vi "DIMPowerSupply.UpdateVoltage.vi"(0 "i ref in":refnum<vi>, 1 "badValue":bool, 2 "moduleValue":dbl format="%.2f", 3 "ms timeout (10000)":i32=10000, 5 "error in (no error)":errorcluster, 6 "voltageQuality":i32) -> (14 "i ref out":refnum<vi>, 17 "timed out":bool, 19 "error out":errorcluster)   [LabVIEW 2014, in "DIMPowerSupply.lvlib"]
doc: "Takes the inpute (raw) voltage and calcutes the real actual voltage [V] delivered by the power supply.\n\nThe value of the actual voltage is written to the attribute data and published via DIM.\n\nThe bad-status bit is also determined and updated."
uses:
  DIMPowerSupply.lvlib
  CSlibraries/UtilityLib/UtilityLib.valueStatus.ctl
  CS_Core/CSApplicationBaseClasses/PSChannelBase/PSChannelBase.statusType.ctl
  CS_Core/CSApplicationBaseClasses/PSChannelBase/PSChannelBase.directionType.ctl
  CS_Core/CSApplicationBaseClasses/PSChannelBase/PSChannelBase.serviceType.ctl
  CS_Core/CSApplicationBaseClasses/PSChannelBase/PSChannelBase.lvlib
  CSlibraries/UtilityLib/UtilityLib.lvlib
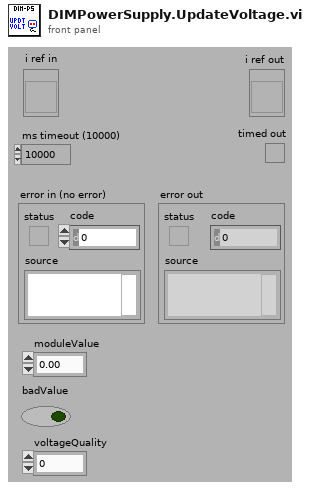
[diagram p1: front panel]
types:
  T1 = typedef "PSChannelBase.lvlib/PSChannelBase.serviceType.ctl" = enum16{"onOff", "voltage", "current", "tripCurrent", "rampUpSpeed", "rampDownSpeed", "status"}
  T2 = typedef "UtilityLib.lvlib/UtilityLib.valueStatus.ctl" = enum16{"no info available", "stand by/off", "on", "warning", "alarm/malfunction", "not implemented", "user action required", "important information", "system default", "control default", "indicator default", "button default"}
  T3 = typedef "PSChannelBase.lvlib/PSChannelBase.directionType.ctl" = enum16{"unknown", "update actual value", "update nominal value", "update both"}
  T4 = typedef "PSChannelBase.lvlib/PSChannelBase.statusType.ctl" = i32
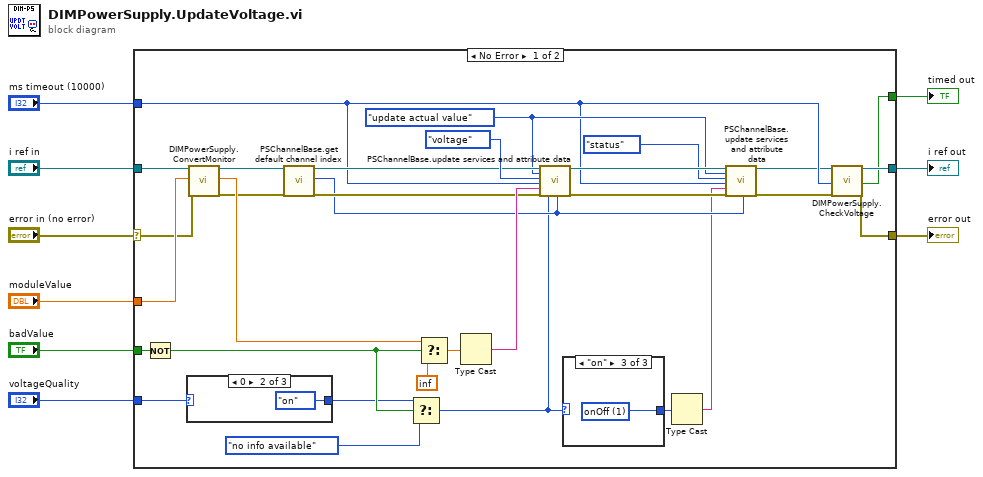
[diagram p0: block diagram]
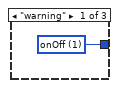
[diagram p2: hidden frame]
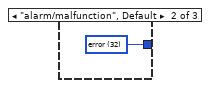
[diagram p3: hidden frame]
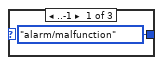
[diagram p4: hidden frame]
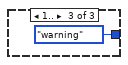
[diagram p5: hidden frame]
diagram:
  n1 = case shown="No Error" "error in (no error)" {
    selector: "error in (no error)" -> [w38 w47]
    tunnel: "i ref in" -> [w40 w48]
    tunnel: "moduleValue" -> [w39 _]
    tunnel: "ms timeout (10000)" -> [w18 _]
    tunnel: [w37 w48] -> w6
    tunnel: [w36 w47] -> w5
    tunnel: [w10 _] -> w4
    tunnel: "badValue" -> [w35 _]
    tunnel: "voltageQuality" -> [w31 _]
    frame No Error {
      w20 = PSChannelBase.directionType."update actual value" ("direction")
      n2 = Not(x=w35) -> (.not. x?=w34:bool)
      n3 = case shown="0" w31 {
        tunnel: [UtilityLib.valueStatus."alarm/malfunction" ("quality") UtilityLib.valueStatus."on" ("quality") UtilityLib.valueStatus."warning" ("quality")] -> w30
        frame ..-1 {
        }
        frame 0 {
        }
        frame 1.. {
        }
      }
      n4 = call "DIMPowerSupply.ConvertMonitor.vi"("i ref in"=w40, "moduleValue"=w39, "error in (no error)"=w38) -> ("i ref out"=w25:refnum<vi>, "actual PS voltage [V]"=w33:dbl, "error out"=w24:errorcluster)  [unwired: 14 in]
      n5 = call "PSChannelBase.get default channel index.vi"("i ref in"=w25, "error in (no error)"=w24) -> ("i ref out"=w23:refnum<vi>, "defaultChannelIndex"=w16:i32, "error out"=w22:errorcluster)  [unwired: 15 in]
      n6 = Select(t=w30, s=w34, f=UtilityLib.valueStatus."no info available" ("quality")) -> (s? t:f=w15:T2)
      n7 = Select(t=w33, s=w34, f=inf ("Positive Infinity")) -> (s? t:f=w27:dbl)
      n8 = Type Cast(x=w27) -> (*(type *) &x=w26:string)  [unwired: 1 in]
      n9 = call "PSChannelBase.update services and attribute data.vi"("i ref in"=w23, "direction"=w20, "service"=PSChannelBase.serviceType."voltage", "ms timeout (10000)"=w18, "value"=w26, "error in (no error)"=w22, "quality"=w15, "channelNumber"=w16) -> ("i ref out"=w21:refnum<vi>, "error out"=w17:errorcluster)  [unwired: 9 in, 1 out]
      n10 = case shown="\"on\"" w15 {
        tunnel: [w41 w42 w43] -> w14
        frame "warning" {
          w41 = T4 1 items=["onOff"=1, "inRange"=2, "rampingUp"=4, "rampingDown"=8, "tripped"=16, "error"=32] ("service")
        }
        frame "alarm/malfunction", Default {
          w42 = T4 32 items=["onOff"=1, "inRange"=2, "rampingUp"=4, "rampingDown"=8, "tripped"=16, "error"=32] ("service")
        }
        frame "on" {
          w43 = T4 1 items=["onOff"=1, "inRange"=2, "rampingUp"=4, "rampingDown"=8, "tripped"=16, "error"=32] ("service")
        }
      }
      n11 = Type Cast(x=w14) -> (*(type *) &x=w13:string)  [unwired: 1 in]
      n12 = call "PSChannelBase.update services and attribute data.vi"("i ref in"=w21, "direction"=w20, "service"=PSChannelBase.serviceType."status", "ms timeout (10000)"=w18, "value"=w13, "error in (no error)"=w17, "channelNumber"=w16) -> ("i ref out"=w12:refnum<vi>, "error out"=w11:errorcluster)  [unwired: 10 in, 1 out]
      n13 = call "DIMPowerSupply.CheckVoltage.vi"("i ref in"=w12, "ms timeout (10000)"=w18, "error in (no error)"=w11) -> ("i ref out"=w37:refnum<vi>, "timed out"=w10:bool, "error out"=w36:errorcluster)  [unwired: 14 in]
    }
    frame Error {
    }
  }
  "error out" <- w5
  "i ref out" <- w6
  "timed out" <- w4
